vi "Example Trigger.vi"() -> ()   [LabVIEW 2015]
uses:
  Input/Input.lvclass
  Result/Result.lvclass
panel:
  out "Error Out":errorcluster
  out "Answer":string
  in  "Greeting":string="Greetings from LabView"
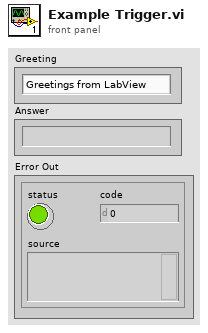
[diagram p1: front panel]
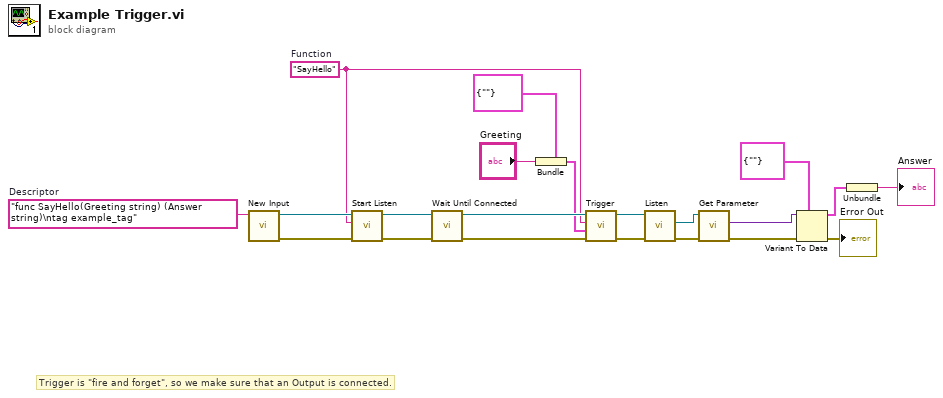
[diagram p0: block diagram]
diagram:
  w18 = "func SayHello(Greeting string) (Answer string)\ntag example_tag"  # Descriptor
  w8 = "SayHello"  # Function
  # "Trigger is \"fire and forget\", so we make sure that an Output is connected."
  n1 = call "New Input.vi"("Descriptor"=w18) -> ("error out"=w13:errorcluster, "input out"=w14:refnum<class "Input.lvclass">)  [unwired: 9 in]
  n2 = call "Start Listen.vi"("error in (no error)"=w13, "Function"=w8, "input in"=w14) -> ("error out"=w11:errorcluster, "input out"=w12:refnum<class "Input.lvclass">)  [unwired: 7 in]
  n3 = call "Wait Until Connected.vi"("error in (no error)"=w11, "input in"=w12) -> ("error out"=w9:errorcluster, "input out"=w10:refnum<class "Input.lvclass">)  [unwired: 7 in, 1 out]
  n4 = Bundle(cluster=cluster{"Greeting":string} {"Greeting"=""}, "Greeting"="Greeting") -> (w7:cluster{"Greeting":string})
  n5 = call "Trigger.vi"("error in (no error)"=w9, "Parameter"=w7, "Function"=w8, "input in"=w10) -> ("error out"=w5:errorcluster, "input out"=w6:refnum<class "Input.lvclass">)  [unwired: 6 in]
  n6 = call-dynamic "Listen.vi"("error in (no error)"=w5, "input in"=w6) -> ("error out"=w1:errorcluster, "Result"=w4:refnum<class "Result.lvclass">)  [unwired: 6 in, 2 out]
  n7 = call-dynamic "Get Parameter.vi"("error in (no error)"=w1, "result in"=w4) -> ("error out"=w2:errorcluster, "Data"=w3:variant)  [unwired: 7 in, 1 out]
  n8 = Variant To Data(error in=w2, type=cluster{"Answer":string} {"Answer"=""}, Variant=w3) -> (data=w19:cluster{"Answer":string}, error out=→"Error Out":errorcluster)
  n9 = Unbundle(w19) -> ("Answer"=→"Answer":string)
